vi "Create Step.vi"(8 "error in (no error)":errorcluster, 9 "Measurement Definition Entry":string, 10 "Measurement Parameters In":refnum<class "String Database.lvclass">, 11 "Measurement Interface in":refnum<class "Measurement Interface.lvclass">) -> (0 "error out":errorcluster, 3 "Measurement Interface out":refnum<class "Measurement Interface.lvclass">)   [LabVIEW 2016, in "Measurement Interface.lvlib" / "Measurement Interface.lvclass"]
uses:
  Measurement Interface.lvclass
  Plugins/String Database.lvlibp/String Database.lvclass
  Measurement Interface.lvclass/Measurement Interface.ctl
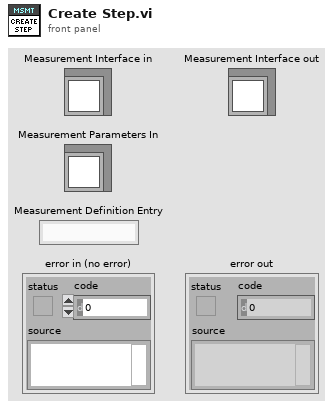
[diagram p1: front panel]
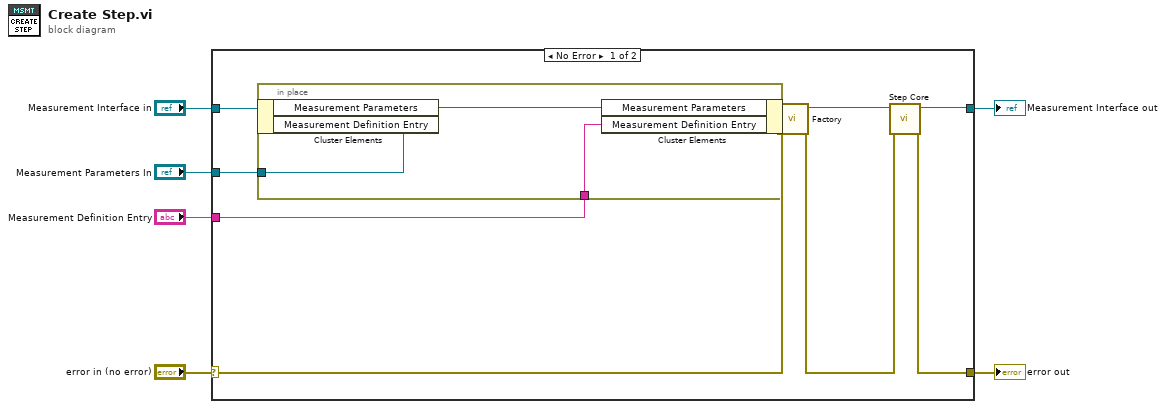
[diagram p0: block diagram]
diagram:
  n1 = case shown="No Error" "error in (no error)" {
    selector: "error in (no error)" -> [w12 w19]
    tunnel: [w10 w19] -> w5
    tunnel: [w8 w18] -> w3
    tunnel: "Measurement Interface in" -> [w15 w18]
    tunnel: "Measurement Parameters In" -> [w14 _]
    tunnel: "Measurement Definition Entry" -> [w7 _]
    frame No Error {
      n2 = in-place {
        in-place-border: w14 -> [w17]
        in-place-border: w7 -> [w16]
        n3 = in-place-cluster #1(w15) -> ()  [unwired: 2 out]
        n4 = in-place-cluster #1("Measurement Parameters"=w17, "Measurement Definition Entry"=w16) -> (w13:refnum<class "Measurement Interface.lvclass">)
      }
      n5 = call-dynamic "Factory.vi"("error in (no error)"=w12, "Measurement Interface in"=w13) -> ("error out"=w11:errorcluster, "Measurement Interface out"=w9:refnum<class "Measurement Interface.lvclass">)  [unwired: 8 in]
      n6 = call-dynamic "Step Core.vi"("error in (no error)"=w11, "Measurement Interface in"=w9) -> ("error out"=w10:errorcluster, "Measurement Interface out"=w8:refnum<class "Measurement Interface.lvclass">)  [unwired: 8 in]
    }
    frame Error {
    }
  }
  "error out" <- w5
  "Measurement Interface out" <- w3
